vi "Global Write.vi"(8 "error in (no error)":errorcluster, 10 "VICI Global":T1, 11 "VISA # in":string) -> (0 "error out":errorcluster, 3 "VISA # out":string)   [LabVIEW 2018, in "VICI M6 M50 Party Mode.lvlib" / "VICI Global Library.lvlib"]
uses:
  VICI Global Library.lvlib
  VICI Global.ctl
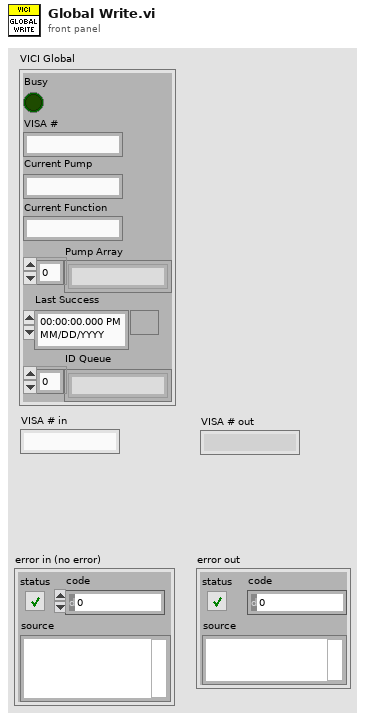
[diagram p1: front panel]
types:
  T1 = typedef "VICI M6 M50 Party Mode.lvlib/VICI Global Library.lvlib/VICI Global.ctl" = cluster{"Busy":bool, "VISA #":string, "Current Pump":string, "Current Function":string, "Pump Array":string[], "Last Success":timestamp, "ID Queue":string[]}
  T2 = cluster{"Busy":bool, "VISA #":string, "Current Pump":string, "Current Function":string, "Pump Array":string[], "Last Success":timestamp, "ID Queue":string[]}[]
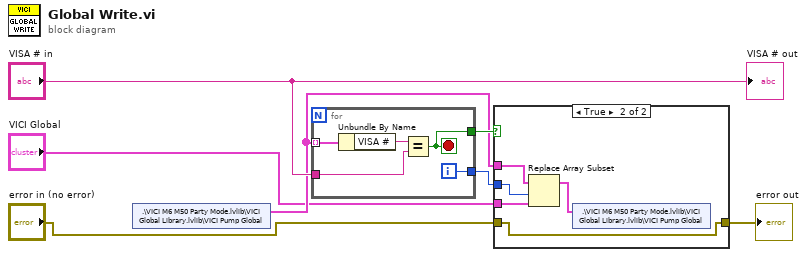
[diagram p0: block diagram]
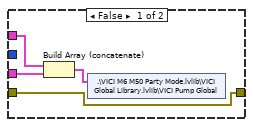
[diagram p2: hidden frame]
diagram:
  n1 = shared-variable ".\\VICI M6 M50 Party Mode.lvlib\\VICI Global Library.lvlib\\VICI Pump Global"() -> (w5:T2)  [unwired: 1 in, 1 out]
  n2 = for {
    tunnel: w5 -> [w12] mode=indexing
    tunnel: "VISA # in" -> [w10]
    tunnel: [w9] -> w3
    tunnel: [w8] -> w6
    i -> [w9]
    stop <- w8 stop-if-true
    n3 = Unbundle By Name(w12) -> ("VISA #"=w11:string)
    n4 = Equal?(x=w11, y=w10) -> (x = y?=w8:bool)
  }
  n5 = case shown="True" w6 {
    tunnel: w5 -> [w16 w20]
    tunnel: "VICI Global" -> [w15 w19]
    tunnel: "error in (no error)" -> [w13 w17]
    tunnel: w3 -> [_ w18]
    tunnel: [w13 w17] -> w2
    frame False {
      n6 = Build Array (concatenate)(w16, w15) -> (w14:T1[])
      n7 = shared-variable ".\\VICI M6 M50 Party Mode.lvlib\\VICI Global Library.lvlib\\VICI Pump Global"(w14) -> ()  [unwired: 1 in, 1 out]
    }
    frame True {
      n8 = Replace Array Subset(array=w20, new element=w19, index=w18) -> (w21:T2)
      n9 = shared-variable ".\\VICI M6 M50 Party Mode.lvlib\\VICI Global Library.lvlib\\VICI Pump Global"(w21) -> ()  [unwired: 1 in, 1 out]
    }
  }
  "error out" <- w2
  "VISA # out" <- "VISA # in"
